vi "Construct by Info Cluster FK Field.vi"(8 "error in (no error)":errorcluster, 10 "FK Ring Info":T1, 11 "FK Ring in":refnum<class "FK Ring.lvclass">) -> (0 "error out":errorcluster, 3 "FK Ring out":refnum<class "FK Ring.lvclass">)   [LabVIEW 2020, in "FK Ring.lvclass"]
uses:
  FK Ring.lvclass
  FK Ring Info.ctl
  FK Ring.lvclass/FK Ring.ctl
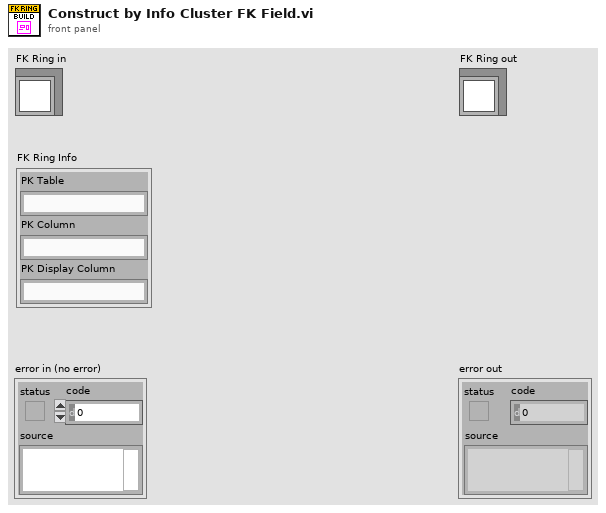
[diagram p1: front panel]
types:
  T1 = typedef "FK Ring Info.ctl" = cluster{"PK Table":string, "PK Column":string, "PK Display Column":string}
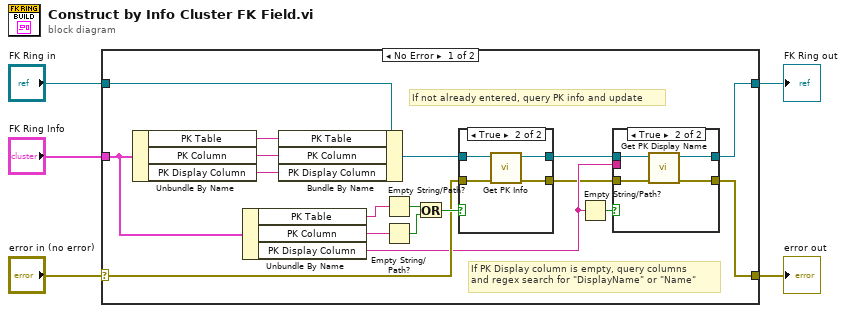
[diagram p0: block diagram]
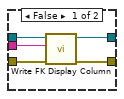
[diagram p2: hidden frame]
diagram:
  n1 = case shown="No Error" "error in (no error)" {
    selector: "error in (no error)" -> [w12 w40]
    tunnel: [w7 w40] -> w4
    tunnel: [w6 w39] -> w2
    tunnel: "FK Ring in" -> [w23 w39]
    tunnel: "FK Ring Info" -> [w17 _]
    frame No Error {
      # "If PK Display column is empty, query columns\nand regex search for \"DisplayName\" or \"Name\""
      # "If not already entered, query PK info and update"
      n2 = Unbundle By Name(w17) -> ("PK Table"=w19:string, "PK Column"=w18:string, "PK Display Column"=w22:string)
      n3 = Unbundle By Name(w17) -> ("PK Table"=w16:string, "PK Column"=w15:string, "PK Display Column"=w9:string)
      n4 = Bundle By Name(cluster=w23, "PK Table"=w19, "PK Column"=w18, "PK Display Column"=w22) -> (w13:refnum<class "FK Ring.lvclass">)
      n5 = Empty String/Path?(string/path=w16) -> (empty?=w21:bool)
      n6 = Empty String/Path?(string/path=w15) -> (empty?=w20:bool)
      n7 = Or(x=w21, y=w20) -> (x .or. y?=w14:bool)
      n8 = case shown="True" w14 {
        tunnel: w13 -> [w34 w38]
        tunnel: w12 -> [w33 w37]
        tunnel: [w33 w36] -> w8
        tunnel: [w34 w35] -> w10
        frame False {
        }
        frame True {
          n9 = call "Get PK Info.vi"("error in (no error)"=w37, "FK Ring in"=w38) -> ("error out"=w36:errorcluster, "FK Ring out"=w35:refnum<class "FK Ring.lvclass">)  [unwired: 8 in]
        }
      }
      n10 = Empty String/Path?(string/path=w9) -> (empty?=w11:bool)
      n11 = case shown="True" w11 {
        tunnel: w10 -> [w28 w32]
        tunnel: w9 -> [w24 _]
        tunnel: w8 -> [w27 w31]
        tunnel: [w26 w30] -> w7
        tunnel: [w25 w29] -> w6
        frame False {
          n12 = call "Write FK Display Column.vi"("error in (no error)"=w27, "PK Display Column"=w24, "FK Ring in"=w28) -> ("error out"=w26:errorcluster, "FK Ring out"=w25:refnum<class "FK Ring.lvclass">)  [unwired: 7 in]
        }
        frame True {
          n13 = call "Get PK Display Name.vi"("error in (no error)"=w31, "FK Ring in"=w32) -> ("error out"=w30:errorcluster, "FK Ring out"=w29:refnum<class "FK Ring.lvclass">)  [unwired: 8 in]
        }
      }
    }
    frame Error {
    }
  }
  "error out" <- w4
  "FK Ring out" <- w2
